vi "Start Main & OCU with Simulator.vi"() -> ()   [LabVIEW 2011]
doc: "Runs the main VI and the OCU on the same computer. simply here for ease of use.\nby Jason Curtis"
uses:
  0-OCU/0 Typedefs/Location of Think.ctl
  1,3 B-Simulation/1,3 B Typedefs/simulator bounds.ctl
  2-Think/2 Typedefs/eStopCommand.ctl
  0-OCU/0 Typedefs/Maps.ctl
panel:
  in  "Map Name":T1="Lake Waban"
  # "running this VI will run OCU and Main on this computer."
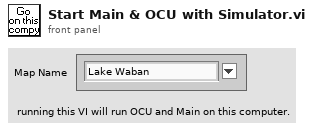
[diagram p1: front panel]
types:
  T1 = typedef "Maps.ctl" = string
  T2 = typedef "eStopCommand.ctl" = enum16{"Reset E-Stop", "Get E-Stop", "Set E-Stop"}
  T3 = typedef "Image Type" = u32
  T4 = typedef "simulator bounds.ctl" = cluster{"Simulator E Range":dbl, "Simulator E Min":dbl, "Simulator N Range":dbl, "Simulator N Min":dbl}
  T5 = typedef "Location of Think.ctl" = string
  T6 = typedef "IMAQ Image.ctl" = refnum<image>
  T7 = typedef "0-Image Descriptor.ctl" = cluster{"Upper-Left Corner Coordinates":T8, "Meters/Pixel":dbl}
  T8 = typedef "UTM Location.ctl" = cluster{"UTM Zone":dbl, "Hemisphere":enum16{"North", "South"}, "East":dbl, "North":dbl}
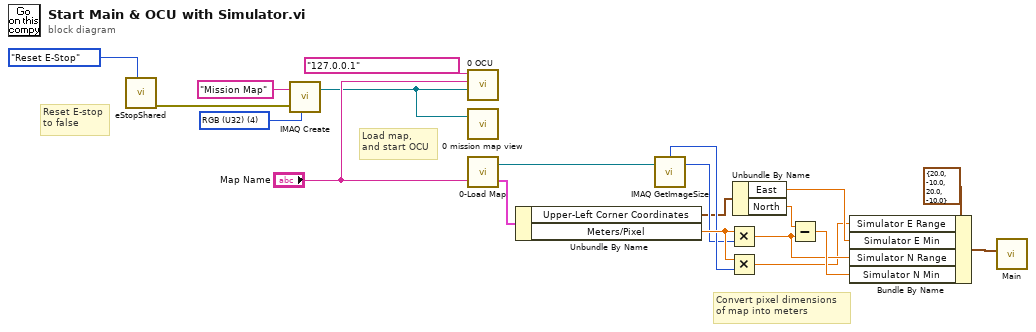
[diagram p0: block diagram]
diagram:
  w5 = T3 4 items=["Grayscale (U8)", "Grayscale (I16)", "Grayscale (SGL)", "Complex (CSG)", "RGB (U32)", "HSL (U32)", "RGB (U64)", "Grayscale (U16)"] ("Image Type")
  # "Load map,\nand start OCU"
  # "Reset E-stop\nto false"
  # "Convert pixel dimensions\nof map into meters"
  n1 = call "eStopShared.vi"("Command"=eStopCommand."Reset E-Stop") -> ("Error Out"=w2:errorcluster)  [unwired: 9 in, 1 out]
  n2 = call "IMAQ Create"("Image Name"="Mission Map", "Image Type"=w5, "error in (no error)"=w2) -> ("New Image"=w1:T6)  [unwired: 1 in, 2 out]
  n3 = call "0 OCU.vi"("Overview Image Ref In"=w1, "Map Name"="Map Name", "Location of THINK"=T5 "127.0.0.1") -> ()  [unwired: 9 in]
  n4 = call "0 mission map view.vi"("Image In"=w1) -> ()  [unwired: 3 in]
  n5 = call "0-Load Map.vi"("Map Name"="Map Name") -> ("Image Descriptor"=w19:T7, "Image Ref Out"=w18:T6)  [unwired: 1 in]
  n6 = Unbundle By Name(w19) -> ("Upper-Left Corner Coordinates"=w13:T8, "Meters/Pixel"=w17:dbl)
  n7 = call "IMAQ GetImageSize"("Image"=w18) -> ("Y Resolution"=w15:i32, "X Resolution"=w16:i32)  [unwired: 3 in, 1 out]
  n8 = Multiply(x=w17, y=w15) -> (x*y=w10:dbl)
  n9 = Multiply(x=w17, y=w16) -> (x*y=w8:dbl)
  n10 = Unbundle By Name(w13) -> ("East"=w9:dbl, "North"=w12:dbl)
  n11 = Subtract(x=w12, y=w10) -> (x-y=w11:dbl)
  n12 = Bundle By Name(cluster=T4 {"Simulator E Range"=20.0, "Simulator E Min"=-10.0, "Simulator N Range"=20.0, "Simulator N Min"=-10.0} ("Simulator Bounds"), "Simulator E Range"=w8, "Simulator E Min"=w9, "Simulator N Range"=w10, "Simulator N Min"=w11) -> (w7:T4)
  n13 = call "Main.vi"("Simulator Bounds"=w7) -> ()  [unwired: 11 in]
